vi "SpawnComponent.vi"(10 "MainCluster":T1, 11 "Component":refnum<class "Actor.lvclass">) -> ()   [LabVIEW 2020, in "jettl.lvlib"]
uses:
  jettl.lvlib
  Actor/Actor.lvclass
  PostSetupCluster.ctl
  MainCluster.ctl
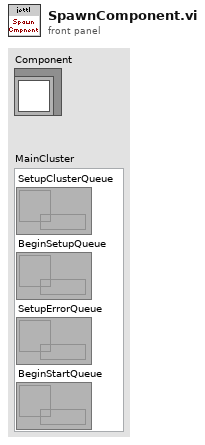
[diagram p1: front panel]
types:
  T1 = typedef "jettl.lvlib/MainCluster.ctl" = cluster{"SetupClusterQueue":refnum<queue>, "BeginSetupQueue":refnum<queue>, "SetupErrorQueue":refnum<queue>, "BeginStartQueue":refnum<queue>}
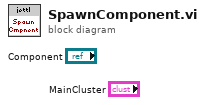
[diagram p0: block diagram]
diagram:
